vi "Write State Machine Status.vi"(8 "error in (no error)":errorcluster, 10 "State Machine Status":T1, 11 "Command State in":refnum<class "State Machine.lvclass">) -> (0 "error out":errorcluster, 3 "Command State out":refnum<class "State Machine.lvclass">)   [LabVIEW 2013, in "State Machine.lvclass"]
uses:
  State Machine.lvclass
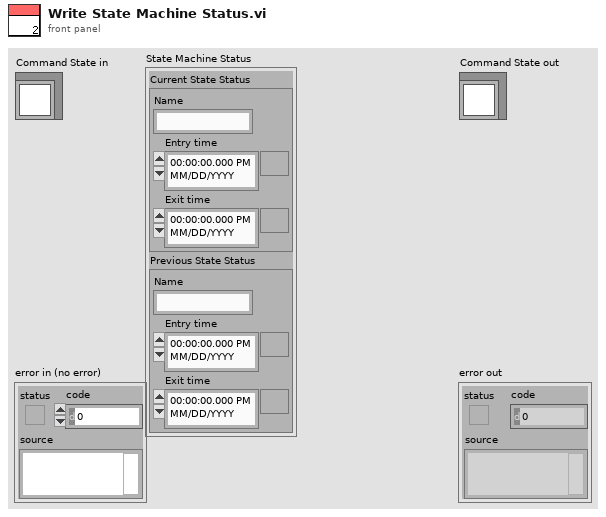
[diagram p1: front panel]
types:
  T1 = cluster{"Current State Status":cluster{"Name":string, "Entry time":timestamp, "Exit time":timestamp}, "Previous State Status":cluster{"Name":string, "Entry time":timestamp, "Exit time":timestamp}}
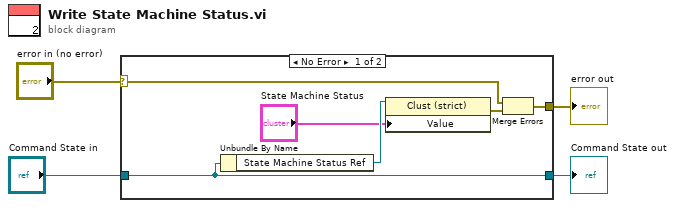
[diagram p0: block diagram]
diagram:
  n1 = case shown="No Error" "error in (no error)" {
    selector: "error in (no error)" -> [w10 w12]
    tunnel: [w6 w12] -> w3
    tunnel: [w9 w11] -> w1
    tunnel: "Command State in" -> [w9 w11]
    frame No Error {
      n2 = Unbundle By Name(w9) -> ("State Machine Status Ref"=w8:refnum<vi>)
      n3 = property class="Clust (strict)"(reference=w8, "Value"="State Machine Status") -> (error out=w5:errorcluster)  [unwired: 1 in, 1 out]
      n4 = Merge Errors(w10, w5) -> (w6:errorcluster)
    }
    frame Error {
    }
  }
  "error out" <- w3
  "Command State out" <- w1
